vi "CalcTemperature.vi"(2 "Temp Voltage (V)":dbl) -> (0 "Temperature (K)":dbl)   [LabVIEW 2016]
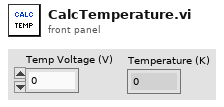
[diagram p1: front panel]
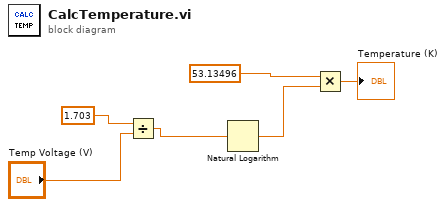
[diagram p0: block diagram]
diagram:
  n1 = Divide(x=1.703, y="Temp Voltage (V)") -> (x/y=w4:dbl)
  n2 = Natural Logarithm(1:w4) -> (0:w2:dbl)
  n3 = Multiply(x=53.13496, y=w2) -> (x*y=→"Temperature (K)":dbl)
